vi "FpgaLink_Check_Nero.vi"(8 "error in (no error)":errorcluster, 11 "handle":i64) -> (0 "error out":errorcluster, 2 "Is Compatible?":bool, 3 "handle out":i64)   [LabVIEW 2011]
doc: "Check to see if the device supports NeroJTAG.\n\nNeroJTAG is a simple JTAG-over-USB protocol, currently implemented for Atmel AVR and Cypress FX2. It uses bulk endpoints 2 and 4. An affirmative response means you can call flPlayXSVF() and flScanChain()."
uses:
  libfpgalink.dll
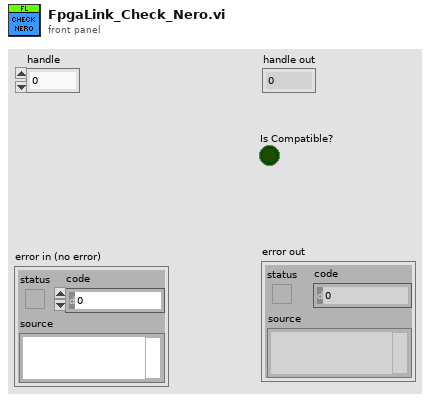
[diagram p1: front panel]
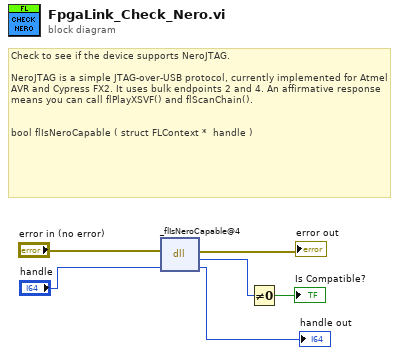
[diagram p0: block diagram]
diagram:
  # "Check to see if the device supports NeroJTAG.\n\nNeroJTAG is a simple JTAG-over-USB protocol, currently implemented for Atmel AVR and Cypress FX2. It uses bulk endpoints 2 and 4. An affirmative response means you can call flPlayXSVF() and flScanChain().\n\n\nbool flIsNeroCapable\t(\tstruct FLContext * \thandle\t)"
  n1 = dll-call lib="libfpgalink.*" fn="_flIsNeroCapable@4"(error in="error in (no error)", "handle"="handle") -> (error out=→"error out":errorcluster, "bool"=w2:u8, "handle"=→"handle out":i64)  [unwired: 2 in, 1 out]
  n2 = Not Equal To 0?(x=w2) -> (x != 0?=→"Is Compatible?":bool)
